vi "DatabaseHand_findSubEle.vi"(9 "name":string, 10 "Data In":T2) -> (1 "found":bool, 2 "Element found":T1, 3 "index":i32)   [LabVIEW 2016]
uses:
  DatabaseHand_Element.ctl
  DatabaseHan_DatabaseElement.ctl
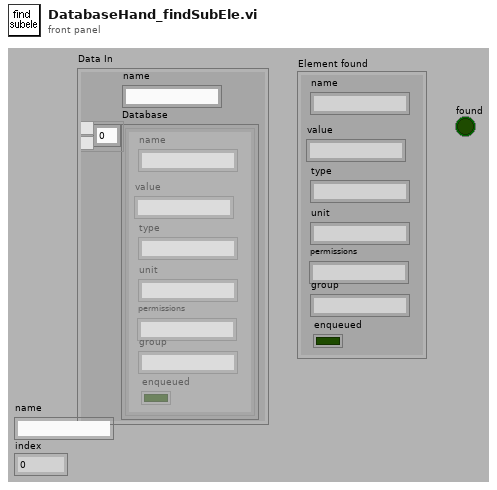
[diagram p1: front panel]
types:
  T1 = typedef "DatabaseHan_DatabaseElement.ctl" = cluster{"name":string, "value":string, "type":string, "unit":string, "permissions":string, "enqueued":bool, "group":string}
  T2 = typedef "DatabaseHand_Element.ctl" = cluster{"name":string, "Database":T1[]}
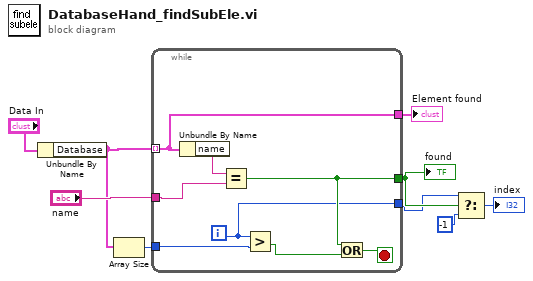
[diagram p0: block diagram]
diagram:
  n1 = Unbundle By Name("Data In") -> ("Database"=w7:T1[])
  n2 = Array Size(array=w7) -> (size(s)=w6:i32)
  n3 = while {
    tunnel: w7 -> [w11] mode=indexing
    tunnel: "name" -> [w16]
    tunnel: w6 -> [w15]
    tunnel: [w12] -> w4
    tunnel: [w11] -> w5
    tunnel: [w10] -> w3
    i -> [w10]
    stop <- w13 stop-if-true
    n4 = Unbundle By Name(w11) -> ("name"=w17:string)
    n5 = Equal?(x=w17, y=w16) -> (x = y?=w12:bool)
    n6 = Greater?(x=w10, y=w15) -> (0:w14:bool)
    n7 = Or(x=w12, y=w14) -> (x .or. y?=w13:bool)
  }
  "Element found" <- w5
  "found" <- w4
  n8 = Select(t=w3, s=w4, f=-1) -> (s? t:f=→"index":i32)
